vi "Example_Mixer.vi"() -> ()   [LabVIEW 2016]
uses:
  WaveIO.dll
panel:
  out "Play Device IDs":i32[](array[numeric])
  out "Play Dev Names":string[](array[string])
  out "# Play Devices":i32
  out "Rec Device IDs":i32[](array[numeric])
  out "Rec Dev Names":string[](array[string])
  out "# Rec Devices":i32
  in  "Part of the Card Name":string
  in  "Find Rec":bool
  in  "Source":u16(ring) items=["Mic", "Line", "Aux", "SPDIF", "HDMI", "Mix", "ANY"]
  in  "Destination":u16(ring) items=["Speaker", "Line", "SPDIF", "HDMI", "ANY"]
  in  "Input Device #":u16
  out "Volume":sgl=50.0 max=100 step=1
  out "Volume":sgl=50.0 max=100 step=1
  in  "Mic Volume":dbl(slide)=52.0 min=0.0 max=100.0 step=0.1 scale=0.0..100.0
  in  "Speaker Volume":dbl(slide)=52.0 min=0.0 max=100.0 step=0.1 scale=0.0..100.0
  out "error out":errorcluster
  in  "Output Device #":u16
  in  "Speaker Mute":bool
  in  "Microphone Mute":bool
  out "Device Names Output":string[](array[string])
  out "Number of Output Devices":i32
  out "Device Names Input":string[](array[string])
  out "Number of Input Devices":i32
  in  "Stop":bool
  # "ONLY for Information Has no effect in the code !"
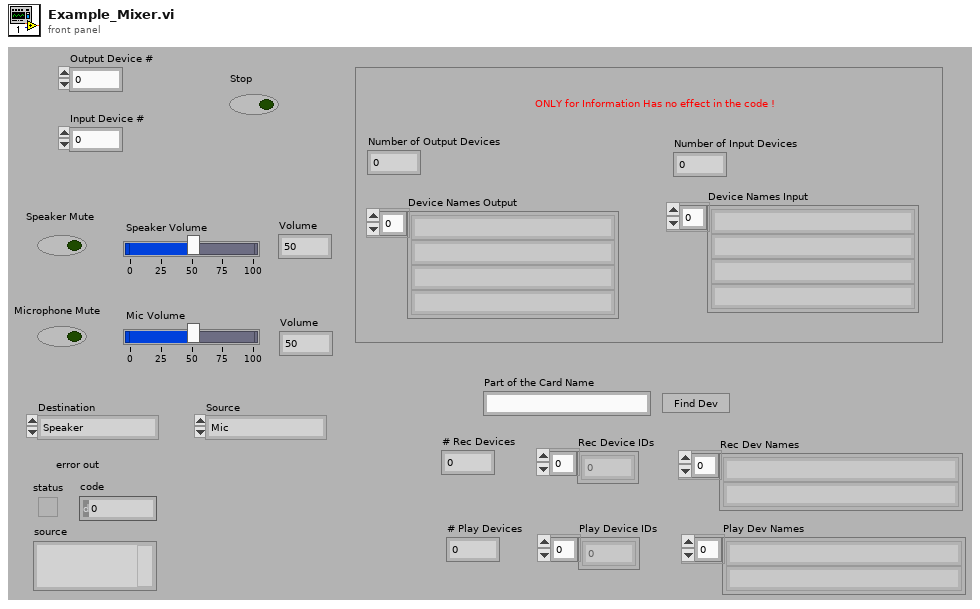
[diagram p1: front panel]
types:
  T1 = enum16{"Set Volume in %", "Set Volume in -dB", "Get volume %", "Get volume dB"}
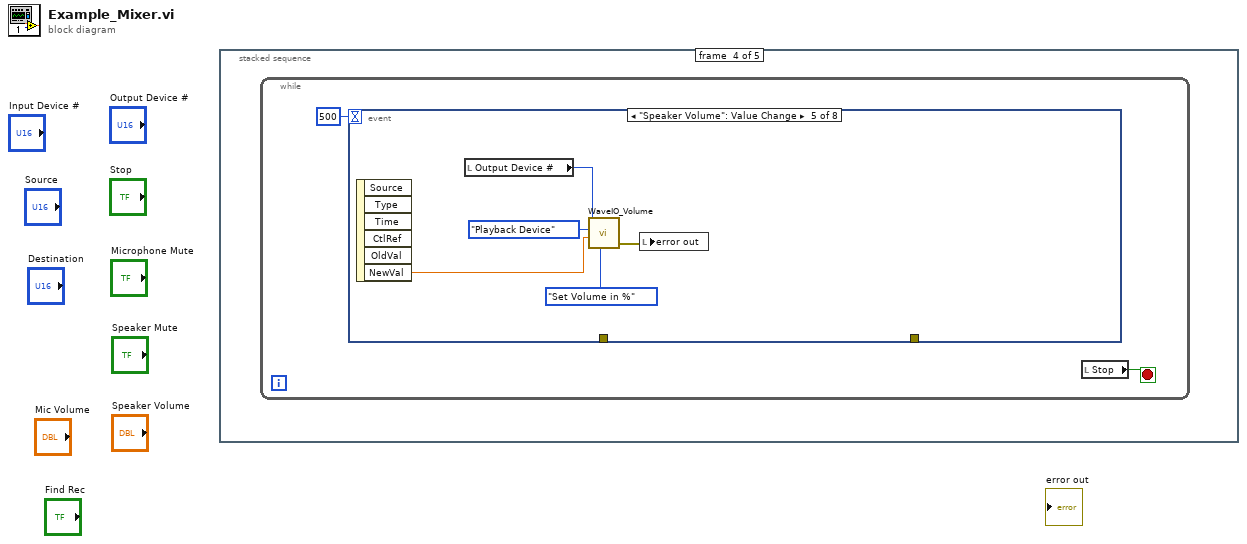
[diagram p0: block diagram]
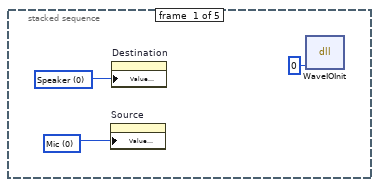
[diagram p2: hidden frame]
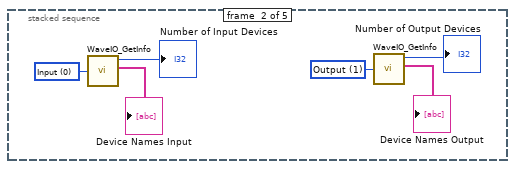
[diagram p3: hidden frame]
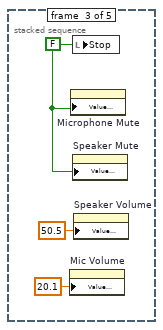
[diagram p4: hidden frame]
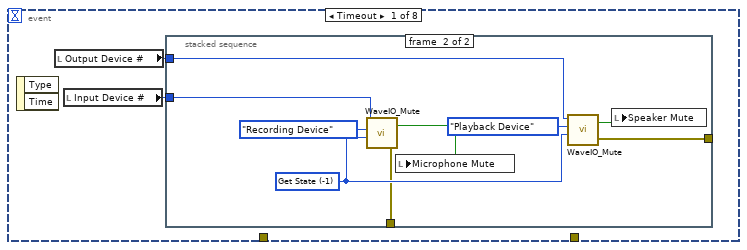
[diagram p5: hidden frame]
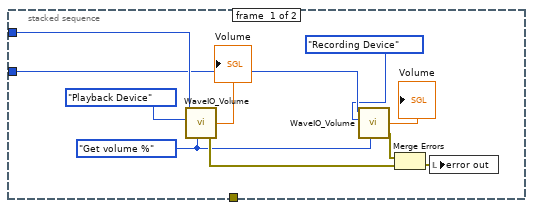
[diagram p6: hidden frame]
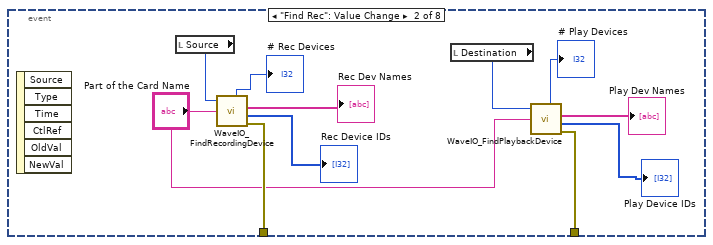
[diagram p7: hidden frame]
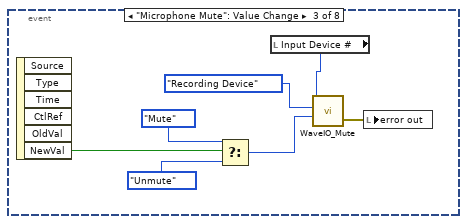
[diagram p8: hidden frame]
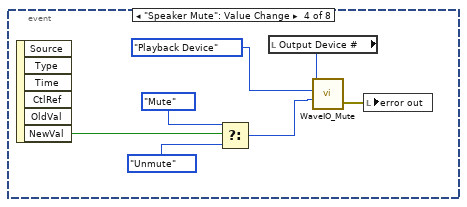
[diagram p9: hidden frame]
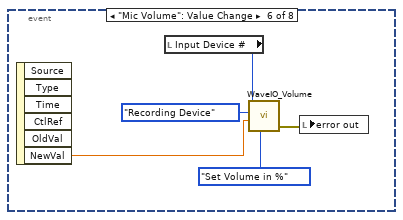
[diagram p10: hidden frame]
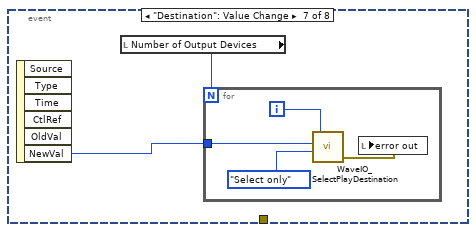
[diagram p11: hidden frame]
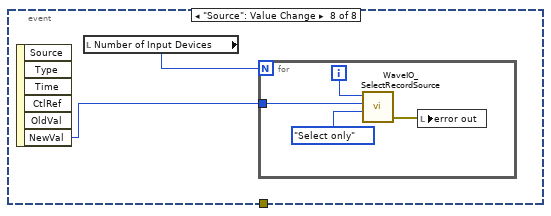
[diagram p12: hidden frame]
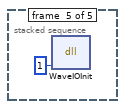
[diagram p13: hidden frame]
diagram:
  n1 = stacked-sequence {
    frame #0 {
      w3 = u16 0 items=["Mic", "Line", "Aux", "SPDIF", "HDMI", "Mix"] ("Source")
      w2 = u16 0 items=["Speaker", "Line", "SPDIF", "HDMI"] ("Destination")
      n2 = property on="Source" class="Ring (strict)"("Value (Signaling)"=w3) -> ()  [unwired: 2 in, 2 out]
      n3 = property on="Destination" class="Ring (strict)"("Value (Signaling)"=w2) -> ()  [unwired: 2 in, 2 out]
      n4 = dll-call lib="D:/Dokumenty/Uczelnia/LabVIEW 2/Lab2 - 09.10.2018/WaveIO/waveio.dll" fn="WaveIOInit"("init"=0) -> ()  [unwired: 5 in, 2 out]
    }
    frame #1 {
      w7 = u16 1 items=["Input", "Output"] ("Direction (Input)")
      w4 = u16 0 items=["Input", "Output"] ("Direction (Input)")
      n5 = call "WaveIO_GetInfo.vi"("Direction (Input)"=w4) -> ("numdev"=→"Number of Input Devices":i32, "Dev Names"=→"Device Names Input":string[])  [unwired: 2 out]
      n6 = call "WaveIO_GetInfo.vi"("Direction (Input)"=w7) -> ("numdev"=→"Number of Output Devices":i32, "Dev Names"=→"Device Names Output":string[])  [unwired: 2 out]
    }
    frame #2 {
      w12 = FALSE ("Stop")
      n7 = property on="Mic Volume" class="Slide (strict)"("Value (Signaling)"=20.1) -> ()  [unwired: 2 in, 2 out]
      n8 = property on="Microphone Mute" class="Bool (strict)"("Value (Signaling)"=w12) -> ()  [unwired: 2 in, 2 out]
      n9 = local write "Stop"(w12) -> ()
      n10 = property on="Speaker Mute" class="Bool (strict)"("Value (Signaling)"=w12) -> ()  [unwired: 2 in, 2 out]
      n11 = property on="Speaker Volume" class="Slide (strict)"("Value (Signaling)"=50.5) -> ()  [unwired: 2 in, 2 out]
    }
    frame #3 {
      n12 = while {
        stop <- w14 stop-if-true
        n13 = event shown="[4] \"Speaker Volume\": Value Change" {
          selector: _ -> [_ _ _ _ _ _ _ _]
          dyn-events: _ -> [_ _ _ _ _ _ _ _]
          timeout: 500 -> [_ _ _ _ _ _ _ _]
          tunnel: [_ w43 _ _ _ _ _ _] -> _
          tunnel: [_ w40 _ _ _ _ _ _] -> _
          event Timeout {
            n14 = event-data() -> ()  [unwired: 1 in, 2 out]
            n15 = local read "Output Device #"() -> (w15:u16)
            n16 = local read "Input Device #"() -> (w16:u16)
            n17 = stacked-sequence {
              tunnel: w16 -> [w24 w35]
              tunnel: w15 -> [w25 w34]
              tunnel: [_ w28] -> _
              tunnel: [_ w27] -> _
              frame #0 {
                w17 = T1."Get volume %" ("Mode")
                n18 = call "WaveIO_Volume.vi"("idev"=w25, "Device type"=enum16{"Recording Device", "Playback Device"}."Playback Device", "Mode"=w17) -> ("Current Volume"=→"Volume":sgl, "error out"=w20:errorcluster)  [unwired: 3 in, 1 out]
                n19 = call "WaveIO_Volume.vi"("idev"=w24, "Device type"=enum16{"Recording Device", "Playback Device"}."Recording Device", "Mode"=w17) -> ("Current Volume"=→"Volume":sgl, "error out"=w19:errorcluster)  [unwired: 3 in, 1 out]
                n20 = Merge Errors(w19, w20) -> (w18:errorcluster)
                n21 = local write "error out"(w18) -> ()
              }
              frame #1 {
                w31 = i16 -1 items=["Unmute"=0, "Mute"=1, "Get State"=-1] ("Flag")
                n22 = call "WaveIO_Mute.vi"("idev"=w35, "Device type"=enum16{"Recording Device", "Playback Device"}."Recording Device", "Flag"=w31) -> ("State"=w33:bool, "error out"=w27:errorcluster)  [unwired: 2 in]
                n23 = local write "Microphone Mute"(w33) -> ()
                n24 = call "WaveIO_Mute.vi"("idev"=w34, "Device type"=enum16{"Recording Device", "Playback Device"}."Playback Device", "Flag"=w31) -> ("State"=w32:bool, "error out"=w28:errorcluster)  [unwired: 2 in]
                n25 = local write "Speaker Mute"(w32) -> ()
              }
            }
          }
          event "Find Rec": Value Change {
            n26 = event-data() -> ()  [unwired: 1 in, 6 out]
            n27 = local read "Source"() -> (w42:u16)
            n28 = call "WaveIO_FindRecordingDevice.vi"("Source"=w42, "Card Name"="Part of the Card Name") -> ("Dev Names"=→"Rec Dev Names":string[], "iDevs"=→"Rec Device IDs":i32[], "error out"=w43:errorcluster, "numdev"=→"# Rec Devices":i32)  [unwired: 1 in, 1 out]
            n29 = local read "Destination"() -> (w36:u16)
            n30 = call "WaveIO_FindPlaybackDevice.vi"("Destination"=w36, "Card Name"="Part of the Card Name") -> ("Dev Names"=→"Play Dev Names":string[], "iDevs"=→"Play Device IDs":i32[], "error out"=w40:errorcluster, "numdev"=→"# Play Devices":i32)  [unwired: 1 in, 1 out]
          }
          event "Microphone Mute": Value Change {
            n31 = event-data() -> ("NewVal"=w52:bool)  [unwired: 1 in, 5 out]
            n32 = Select(t=enum16{"Unmute", "Mute", "Get State"}."Mute" ("Flag"), s=w52, f=enum16{"Unmute", "Mute", "Get State"}."Unmute" ("Flag")) -> (s? t:f=w49:enum16{"Unmute", "Mute", "Get State"})
            n33 = local read "Input Device #"() -> (w48:u16)
            n34 = call "WaveIO_Mute.vi"("idev"=w48, "Device type"=enum16{"Recording Device", "Playback Device"}."Recording Device", "Flag"=w49) -> ("error out"=w53:errorcluster)  [unwired: 2 in, 1 out]
            n35 = local write "error out"(w53) -> ()
          }
          event "Speaker Mute": Value Change {
            n36 = event-data() -> ("NewVal"=w58:bool)  [unwired: 1 in, 5 out]
            n37 = Select(t=enum16{"Unmute", "Mute", "Get State"}."Mute" ("Flag"), s=w58, f=enum16{"Unmute", "Mute", "Get State"}."Unmute" ("Flag")) -> (s? t:f=w55:enum16{"Unmute", "Mute", "Get State"})
            n38 = local read "Output Device #"() -> (w60:u16)
            n39 = call "WaveIO_Mute.vi"("idev"=w60, "Device type"=enum16{"Recording Device", "Playback Device"}."Playback Device", "Flag"=w55) -> ("error out"=w59:errorcluster)  [unwired: 2 in, 1 out]
            n40 = local write "error out"(w59) -> ()
          }
          event "Speaker Volume": Value Change {
            n41 = event-data() -> ("NewVal"=w64:dbl)  [unwired: 1 in, 5 out]
            n42 = local read "Output Device #"() -> (w65:u16)
            n43 = call "WaveIO_Volume.vi"("idev"=w65, "Device type"=enum16{"Recording Device", "Playback Device"}."Playback Device", "Volume"=w64, "Mode"=T1."Set Volume in %") -> ("error out"=w63:errorcluster)  [unwired: 2 in, 2 out]
            n44 = local write "error out"(w63) -> ()
          }
          event "Mic Volume": Value Change {
            n45 = event-data() -> ("NewVal"=w70:dbl)  [unwired: 1 in, 5 out]
            n46 = local read "Input Device #"() -> (w68:u16)
            n47 = call "WaveIO_Volume.vi"("idev"=w68, "Device type"=enum16{"Recording Device", "Playback Device"}."Recording Device", "Volume"=w70, "Mode"=T1."Set Volume in %") -> ("error out"=w69:errorcluster)  [unwired: 2 in, 2 out]
            n48 = local write "error out"(w69) -> ()
          }
          event "Destination": Value Change {
            n49 = event-data() -> ("NewVal"=w72:u16)  [unwired: 1 in, 5 out]
            n50 = local read "Number of Output Devices"() -> (w71:i32)
            n51 = for {
              N: w71 -> [_]
              tunnel: w72 -> [w76]
              i -> [w73]
              n52 = call "WaveIO_SelectPlayDestination.vi"("Mode"=enum16{"Select only", "Select/Unmut/Vol=100%"}."Select only", "Destination"=w76, "idev"=w73) -> ("error out"=w75:errorcluster)  [unwired: 2 in, 1 out]
              n53 = local write "error out"(w75) -> ()
            }
          }
          event "Source": Value Change {
            n54 = event-data() -> ("NewVal"=w78:u16)  [unwired: 1 in, 5 out]
            n55 = local read "Number of Input Devices"() -> (w77:i32)
            n56 = for {
              N: w77 -> [_]
              tunnel: w78 -> [w82]
              i -> [w79]
              n57 = call "WaveIO_SelectRecordSource.vi"("Mode"=enum16{"Select only", "Select/Unmut/Vol=100%"}."Select only", "Source"=w82, "idev"=w79) -> ("error out"=w81:errorcluster)  [unwired: 2 in, 1 out]
              n58 = local write "error out"(w81) -> ()
            }
          }
        }
        n59 = local read "Stop"() -> (w14:bool)
      }
    }
    frame #4 {
      n60 = dll-call lib="D:/Dokumenty/Uczelnia/LabVIEW 2/Lab2 - 09.10.2018/WaveIO/waveio.dll" fn="WaveIOInit"("init"=1) -> ()  [unwired: 5 in, 2 out]
    }
  }
